vi "SC TCP SoundCheck Wait for Ready.vi"(7 "TimeOut(s)":dbl=2.0, 8 "error in (no error)":errorcluster, 10 "port (4444)":u16=4444, 11 "SoundCheck IP Address (localhost)":string="localhost") -> (0 "error out":errorcluster, 2 "Duration":dbl, 3 "Ready":bool)   [LabVIEW 2018]
doc: "Allows the user to control the running of a SoundCheck sequence from their own LabVIEW application."
uses:
  Common/Utils/Errors/Error.Error Code List.ctl
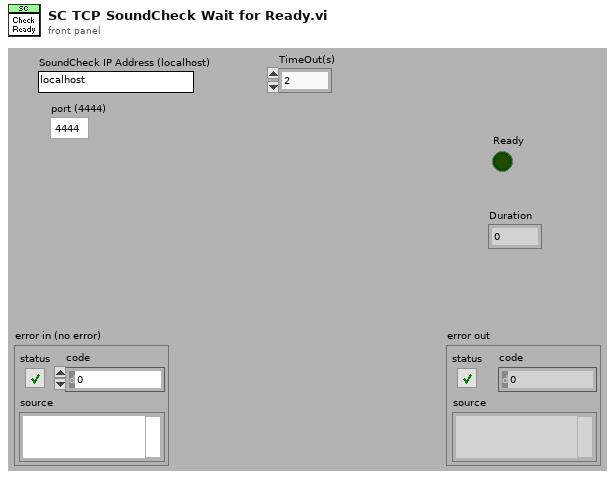
[diagram p1: front panel]
types:
  T1 = typedef "Error.Error Code List.ctl" = i32
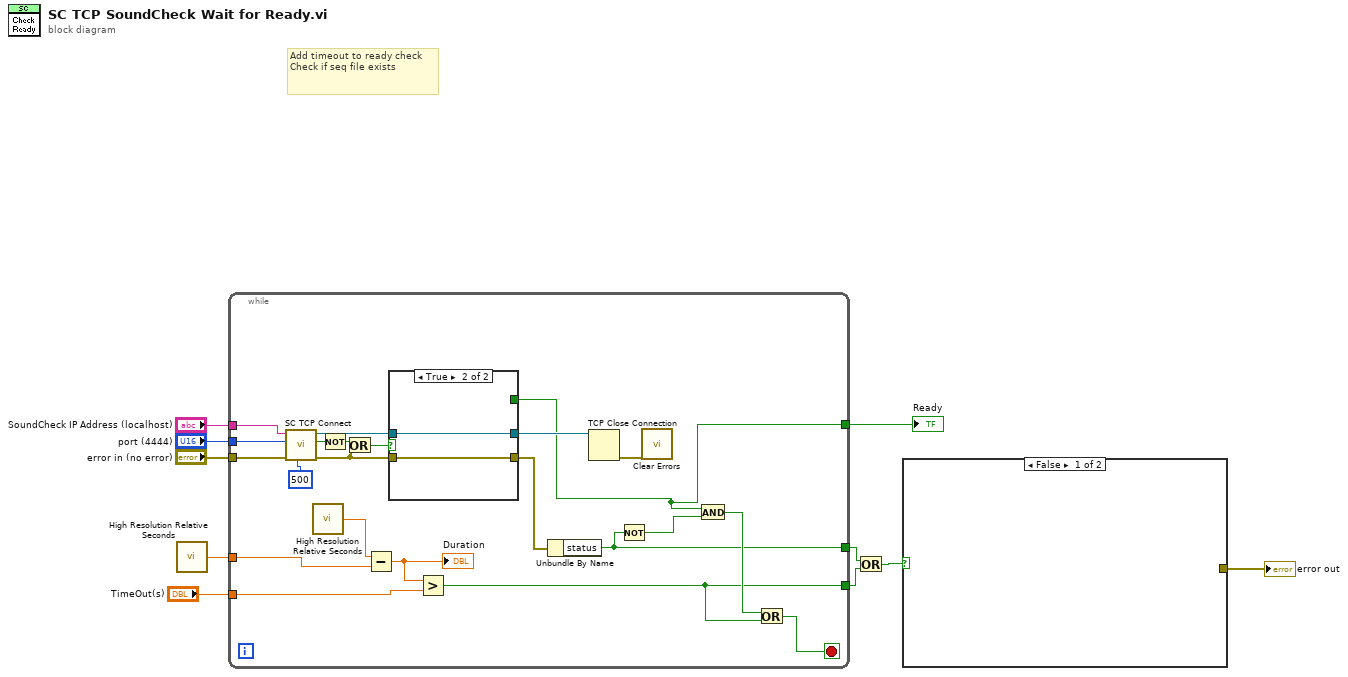
[diagram p0: block diagram]
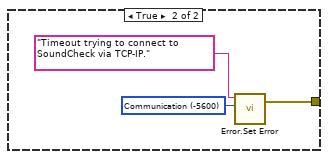
[diagram p2: hidden frame]
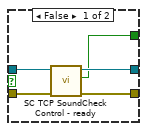
[diagram p3: hidden frame]
diagram:
  # "Add timeout to ready check\nCheck if seq file exists"
  n1 = call <vilib>:"High Resolution Relative Seconds.vi"() -> ("relative seconds"=w7:dbl)
  n2 = while {
    tunnel: "error in (no error)" -> [w32]
    tunnel: "SoundCheck IP Address (localhost)" -> [w31]
    tunnel: "port (4444)" -> [w30]
    tunnel: w7 -> [w17]
    tunnel: "TimeOut(s)" -> [w15]
    tunnel: [w13] -> w5
    tunnel: [w12] -> w4
    tunnel: [w11] -> w1
    stop <- w14 stop-if-true
    n3 = call "SC TCP Connect.vi"("timeout ms (10000)"=500, "error in (no error)"=w32, "port"=w30, "Server IP Address"=w31) -> ("error out"=w27:errorcluster, "Connected"=w28:bool, "TCP Network Connection out"=w29:refnum<k5>)  [unwired: 5 in]
    n4 = call <vilib>:"High Resolution Relative Seconds.vi"() -> ("relative seconds"=w18:dbl)
    n5 = Not(x=w28) -> (.not. x?=w25:bool)
    n6 = Or(x=w25, y=w27) -> (x .or. y?=w26:bool)
    n7 = Subtract(x=w18, y=w17) -> (x-y=w16:dbl)
    "Duration" <- w16
    n8 = case shown="True" w26 {
      tunnel: [w34 w41] -> w21
      tunnel: w29 -> [w36 w43]
      tunnel: w27 -> [w37 w42]
      tunnel: [w35 w43] -> w24
      tunnel: [w33 _] -> w11
      frame False {
        n9 = call "SC TCP SoundCheck Control - ready.vi"("error in (no error)"=w37, "connection ID in"=w36) -> ("error out"=w34:errorcluster, "ready?"=w33:bool, "connection ID out"=w35:refnum<k5>)  [unwired: 7 in]
      }
      frame True {
        w38 = T1 -5600 items=["No Error"=0, "Abort"=-2, "Misc"=-5000, "Fixture Error"=-5100, "File IO - General"=-5200, "FIle IO - Config Error"=-5201, "Instrument - General"=-5300, "Instrument - Serial Com"=-5301, "Instrument - Camera"=-5302, "Instrument - PS"=-5303, "Instrument - Oscilloscope"=-5304, "Instrument - Function Gen"=-5305, "Instrument - Load"=-5306, "Instrument - Meter"=-5307, "Instrument - Power Control"=-5308, "Instrument - Motion"=-5309, "Instrument - RF"=-5310, "System Exe"=-5400, "Image Processing"=-5500, "Communication"=-5600, "Script - Syntax Error"=-6000, "Script - Invalid Name or Param"=-6100, "Script - Timeout"=-6200, "Invalid Data"=-6300, "FW Update Error"=-6500] ("Std Code")
        n10 = call "Error.Set-Change Error Info.vi"("Std Code"=w38, "error in"=w42, "Description"="Failed to connect to the SoundCheck application over TCP-IP.", "Set Error"=TRUE) -> ("error out"=w41:errorcluster)  [unwired: 7 in]
      }
    }
    n11 = Greater?(x=w16, y=w15) -> (0:w12:bool)
    n12 = Unbundle By Name(w21) -> ("status"=w13:bool)
    n13 = TCP Close Connection(connection ID=w24) -> (error out=w22:errorcluster)  [unwired: 2 in, 1 out]
    n14 = Not(x=w13) -> (.not. x?=w20:bool)
    n15 = call <vilib>:"Clear Errors.vi"("error in (no error)"=w22) -> ()  [unwired: 5 in, 2 out]
    n16 = And(x=w11, y=w20) -> (x .and. y?=w19:bool)
    n17 = Or(x=w19, y=w12) -> (x .or. y?=w14:bool)
  }
  "Ready" <- w1
  n18 = Or(x=w5, y=w4) -> (x .or. y?=w3:bool)
  n19 = case shown="False" w3 {
    tunnel: [_ w44] -> w2
    frame False {
    }
    frame True {
      w45 = T1 -5600 items=["No Error"=0, "Abort"=-2, "Misc"=-5000, "Fixture Error"=-5100, "File IO - General"=-5200, "FIle IO - Config Error"=-5201, "Instrument - General"=-5300, "Instrument - Serial Com"=-5301, "Instrument - Camera"=-5302, "Instrument - PS"=-5303, "Instrument - Oscilloscope"=-5304, "Instrument - Function Gen"=-5305, "Instrument - Load"=-5306, "Instrument - Meter"=-5307, "Instrument - Power Control"=-5308, "Instrument - Motion"=-5309, "Instrument - RF"=-5310, "System Exe"=-5400, "Image Processing"=-5500, "Communication"=-5600, "Script - Syntax Error"=-6000, "Script - Invalid Name or Param"=-6100, "Script - Timeout"=-6200, "Invalid Data"=-6300, "FW Update Error"=-6500] ("Std Code")
      n20 = call "Error.Set Error.vi"("Code"=w45, "Desc"="Timeout trying to connect to SoundCheck via TCP-IP.") -> ("error out"=w44:errorcluster)  [unwired: 5 in]
    }
  }
  "error out" <- w2
